vi "Calibrate Polarizer.vi"(8 "error in (no error)":errorcluster, 11 "Thorlabs Polarizer.lvlib:Thorlabs Polarizer.lvclass 2":refnum<class "Thorlabs Polarizer.lvclass">) -> (0 "error out":errorcluster, 3 "Thorlabs Polarizer.lvlib:Thorlabs Polarizer.lvclass":refnum<class "Thorlabs Polarizer.lvclass">)   [LabVIEW 2023, in "Thorlabs Polarizer.lvlib" / "Thorlabs Polarizer.lvclass"]
uses:
  Thorlabs Polarizer.lvclass
  Thorlabs Polarizer.lvclass/Thorlabs Polarizer.ctl
  Thorlabs Polarizer.lvlib
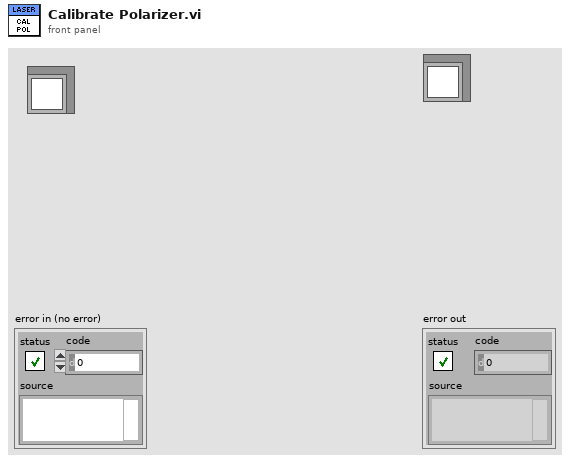
[diagram p1: front panel]
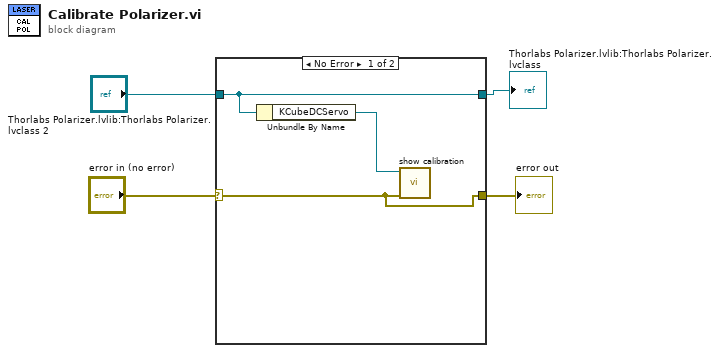
[diagram p0: block diagram]
diagram:
  n1 = case shown="No Error" "error in (no error)" {
    selector: "error in (no error)" -> [w5 w9]
    tunnel: [w5 w9] -> w3
    tunnel: [w7 w8] -> w1
    tunnel: "Thorlabs Polarizer.lvlib:Thorlabs Polarizer.lvclass 2" -> [w7 w8]
    frame No Error {
      n2 = Unbundle By Name(w7) -> ("KCubeDCServo"=w6:refnum<k24>)
      n3 = call "show calibration.vi"("error in"=w5, "KCubeDCServo"=w6) -> ()  [unwired: 4 in, 4 out]
    }
    frame Error {
    }
  }
  "error out" <- w3
  "Thorlabs Polarizer.lvlib:Thorlabs Polarizer.lvclass" <- w1
